vi "get adc volt.vi"(8 "error in (no error)":errorcluster, 11 "ch":i32) -> (0 "error out":errorcluster, 3 "function return":sgl)   [LabVIEW 2014, in "libroboticscape.lvlib"]
doc: "float get_adc_volt(int ch);"
uses:
  libroboticscape.lvlib
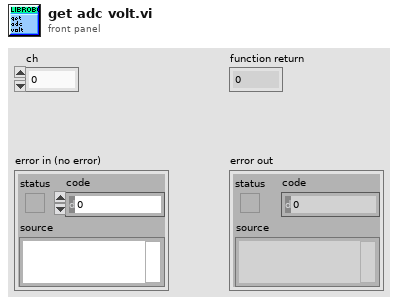
[diagram p1: front panel]
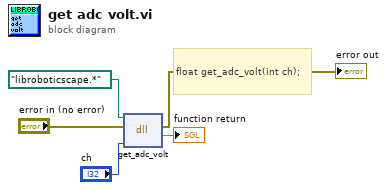
[diagram p0: block diagram]
diagram:
  # "float get_adc_volt(int ch);"
  n1 = dll-call lib="C:/Users/ktalke/Documents/Robotics-Cape-Master-Jessie/Libroboticscape-Master-Jessie/libroboticscape.so" fn="get_adc_volt"(path in=path "libroboticscape.*", error in="error in (no error)", "ch"="ch") -> (error out=→"error out":errorcluster, "return type"=→"function return":sgl)  [unwired: 2 in, 1 out]
